vi "Global - Configuration Options.vi"() -> ()   [LabVIEW 2013]
panel:
  in  "Error Log Path":path=path "c:/log/log.txt" caption="错误记录路径"
  in  "Data Log Folder":path=path "C:/data" caption="数据记录文件夹"
  in  "Network Stream Buffer Size":i32=50 caption="网络流缓冲区大小"
  in  "Reboot Timestamp Log":path=path "c:/log/reboots.txt" caption="重启时间标识记录"
  in  "Error Log Duplicate Interval (ms)":u32=5000 caption="错误记录重复间隔（毫秒）"
  in  "Network Stream Polling Timeout (ms)":i32=500 caption="网络流轮询超时（毫秒）"
  in  "Debugging":bool=TRUE caption="调试"
  in  "Error Log Max Size (bytes)":i64=100000 caption="错误记录最大大小（字节）"
  in  "RT Stream Name":string="RT发出的命令流" caption="RT流名称"
  in  "Monitoring Loop Rate (ms)":u32=200 caption="监测循环频率（毫秒）"
  in  "UI Stream Name":string="UI发出的命令流" caption="UI流名称"
  in  "Network Stream Connect Timeout (ms)":i32=5000 caption="网络流连接超时（毫秒）"
  # "如果修改了任何默认配置选项，必须在保存本VI之前选择编辑>>当前值设为默认值。"
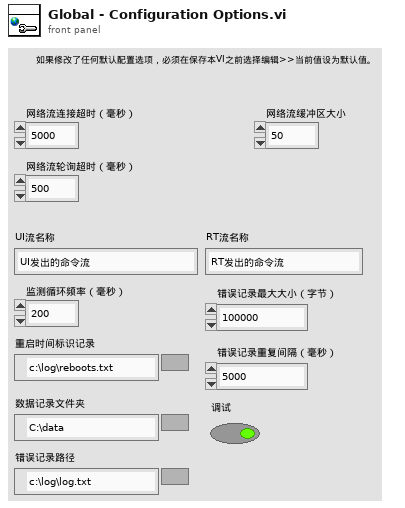
[diagram p1: front panel]
diagram:
